vi "WriteAndRead.vi"(8 "error in (no error)":errorcluster, 10 "Data":u8[](array[numeric])=[0], 11 "PCA in":refnum<class "PCA.lvclass">) -> (0 "error out":errorcluster, 2 "Data 2":u8[](array[numeric]), 3 "PCA out":refnum<class "PCA.lvclass">)   [LabVIEW 2022 SP3, in "PCA9685.lvlib" / "PCA.lvclass"]
uses:
  PCA.lvclass
  <vilib>/MakerHub/LINX/Private/Type Defs/Peripherals/I2C/EOF.ctl
  PCA.lvclass/PCA.ctl
  <vilib>/MakerHub/LINX/Private/Local IO/LinxI2cWrite.vi
  <vilib>/MakerHub/LINX/Public/Utilities/Check Channel.vi
  <vilib>/MakerHub/LINX/Private/Local IO/Handle Errors.vi
  <vilib>/MakerHub/LINX/Private/Utilties/Generate Error.vi
  <vilib>/MakerHub/LINX/LMH-LINX.lvlib
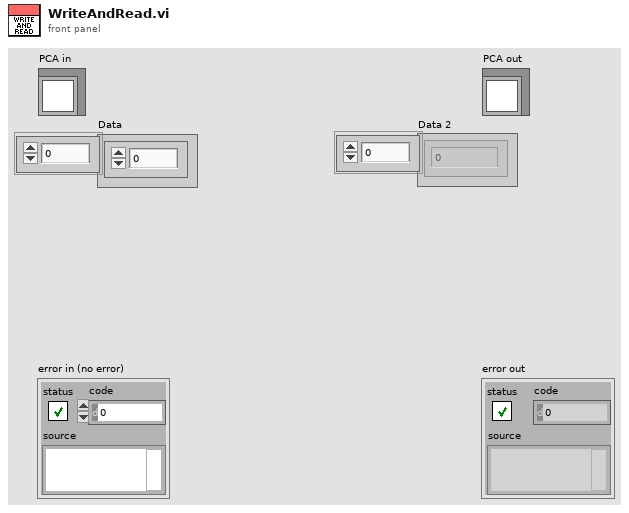
[diagram p1: front panel]
types:
  T1 = typedef "LMH-LINX.lvlib/EOF.ctl" = enum8{"Stop", "Restart", "Restart No Stop", "No Stop"}
  T2 = typedef "PCA9685.lvlib/PCA.lvclass/LinxI2C.ctl" = cluster{"I2C Slave Address (0)":u16, "I2C Chanel":u16, "LINX Resource":T3}
  T3 = typedef "LMH-LINX.lvlib/LINX Ref.ctl" = cluster{"IO":T4, "Interface":T5, "LINX Device Config":T6}
  T4 = typedef "LMH-LINX.lvlib/Platform.ctl" = enum16{"Remote", "Local"}
  T5 = typedef "LMH-LINX.lvlib/Interface.ctl" = enum16{"Serial", "TCP"}
  T6 = typedef "LMH-LINX.lvlib/Device.lvlib/LINX Device Config.ctl" = cluster{"Interface":T5, "COM Port":refnum<visa-resource-name>, "TCP Configuration":T7, "Device Family":u8, "Device ID":u8, "Device Name":string, "TCP Ref":refnum<k5>, "Channels":T8}
  T7 = typedef "LMH-LINX.lvlib/Device.lvlib/TCP Config.ctl" = cluster{"IP Address":string, "Port":u16}
  T8 = typedef "LMH-LINX.lvlib/Channels.ctl" = cluster{"DI":u8[], "DO":u8[], "AI":u8[], "AO":u8[], "PWM":u8[], "QE":u8[], "UART":u8[], "I2C 2":u8[], "SPI":u8[], "CAN":u8[], "Servo":u8[], "AI Ref (V)":dbl, "AI Resolution (Bits)":u8, "AO Ref (V)":dbl, "AO Resolution (Bits)":u8}
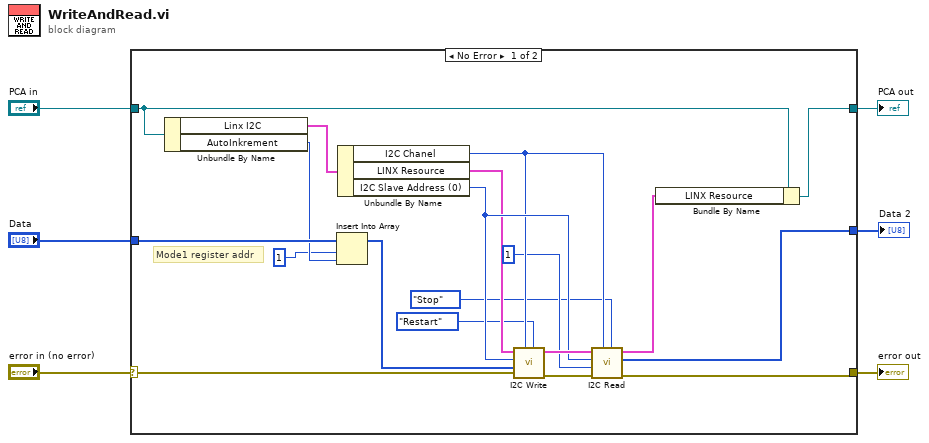
[diagram p0: block diagram]
diagram:
  n1 = case shown="No Error" "error in (no error)" {
    selector: "error in (no error)" -> [w18 w27]
    tunnel: [w16 w27] -> w5
    tunnel: [w23 w26] -> w3
    tunnel: "PCA in" -> [w24 w26]
    tunnel: "Data" -> [w10 _]
    tunnel: [w14 _] -> w1
    frame No Error {
      # "Mode1 register addr"
      n2 = Unbundle By Name(w24) -> ("Linx I2C"=w25:T2, "AutoInkrement"=w9:u8)
      n3 = Insert Into Array(array=w10, index=u8 1 ("Mode1.AutoInkrement"), new element=w9) -> (w7:u8[])
      n4 = Unbundle By Name(w25) -> ("I2C Chanel"=w19:u16, "LINX Resource"=w20:T3, "I2C Slave Address (0)"=w21:u16)
      n5 = call <vilib>:"I2C Write.vi"("EOF"=EOF."Restart", "I2C Channel"=w19, "Error In"=w18, "Data"=w7, "I2C Slave Address (0)"=w21, "LINX Resource"=w20) -> ("Error Out"=w17:errorcluster, "LINX Resource"=w22:T3)  [unwired: 4 in]
      n6 = call <vilib>:"I2C Read.vi"("EOF"=EOF."Stop", "I2C Channel"=w19, "Error In"=w17, "Bytes To Read"=u8 1, "I2C Slave Address (0)"=w21, "LINX Resource"=w22) -> ("Error Out"=w16:errorcluster, "Data"=w14:u8[], "LINX Resource"=w15:T3)  [unwired: 3 in]
      n7 = Bundle By Name(cluster=w24, "LINX Resource"=w15) -> (w23:refnum<class "PCA.lvclass">)
    }
    frame Error {
    }
  }
  "error out" <- w5
  "PCA out" <- w3
  "Data 2" <- w1
